vi "AddProjectLibrary.vi"(8 "error in (no error)":errorcluster, 10 "Path":path, 11 "TestSuite in":refnum<class "TestSuite.lvclass">) -> (0 "error out":errorcluster, 3 "TestSuite out":refnum<class "TestSuite.lvclass">)   [LabVIEW 2019, in "TestSuite.lvclass"]
uses:
  TestSuite.lvclass
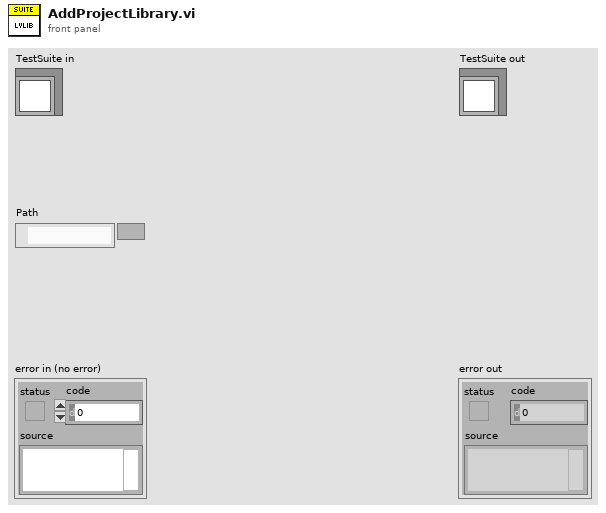
[diagram p1: front panel]
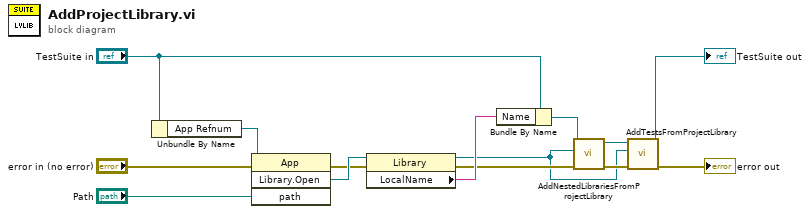
[diagram p0: block diagram]
diagram:
  n1 = Unbundle By Name("TestSuite in") -> ("App Refnum"=w12:refnum<vi>)
  n2 = invoke class="App" method="Library.Open"(reference=w12, error in="error in (no error)", "path"="Path") -> (error out=w10:errorcluster, "Open Library"=w11:refnum<vi>)  [unwired: 1 in, 2 out]
  n3 = property class="Library"(reference=w11, error in=w10) -> (reference out=w1:refnum<vi>, error out=w5:errorcluster, "LocalName"=w8:string)
  n4 = Bundle By Name(cluster="TestSuite in", "Name"=w8) -> (w2:refnum<class "TestSuite.lvclass">)
  n5 = call "AddNestedLibrariesFromProjectLibrary.vi"("error in (no error)"=w5, "Library"=w1, "TestSuite in"=w2) -> ("error out"=w4:errorcluster, "TestSuite out"=w3:refnum<class "TestSuite.lvclass">)  [unwired: 7 in]
  n6 = call "AddTestsFromProjectLibrary.vi"("error in (no error)"=w4, "Library"=w1, "TestSuite in"=w3) -> ("error out"=→"error out":errorcluster, "TestSuite out"=→"TestSuite out":refnum<class "TestSuite.lvclass">)  [unwired: 7 in]
